vi "MetronomeCreate.vi"() -> (3 "Metronome.lvclass":refnum<class "Metronome.lvclass">)   [LabVIEW 2019, in "Metronome.lvclass"]
uses:
  Metronome.lvclass
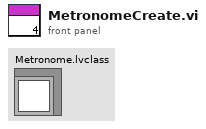
[diagram p1: front panel]
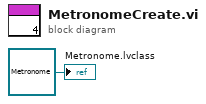
[diagram p0: block diagram]
diagram:
  "Metronome.lvclass" <- refnum<class "Metronome.lvclass"> refnum ("Metronome.lvclass")
